vi "Config Input Type.vi"(0 "VISA resource name":refnum<visa-resource-name>, 1 "Sensor Type (0: Special)":i8(ring) items=["Special", "Silicon Diode", "GaAIAS Diode", "Platinum 100 (250 Ohm)", "Platinum 100 (500 Ohm)", "Platinum 1000", "Rhodium Iron", "Carbon Glass", "Cernox", "RuOx", "Germanium"], 2 "Coefficient (0: None)":i8(ring) items=["None", "Negative", "Positive"], 5 "Input (0: A)":u16(ring) items=["A", "B", "C", "D"], 7 "Units (0: None)":i8(ring) items=["None", "Volts", "Ohms"], 9 "Excitation (0: None)":i8(ring), 11 "error in (no error)":errorcluster, 12 "Range (0: None)":i8(ring) items=["None", "1mV", "2.5mV", "5mV", "10mV", "25mV", "50mV", "100mV", "250mV", "500mV", "1V", "2.5V", "5V", "7V"]) -> (4 "VISA resource name out":refnum<visa-resource-name>, 15 "error out":errorcluster)   [LabVIEW 2019, in "Lake Shore Cryotronics 340.lvlib"]
doc: "This VI configures the following parameters for a 340 input's type:\nSensor Type, Units, Coefficient, Excitation, and Range.\nNote that if Sensor Type is not special, none of the other parameters will not be sent as they are pre-determined by this instrument.\nThe LSCI 340 Status - Busy.vi should be used after this vi to verify the instrument has finished processing the commands."
uses:
  Lake Shore Cryotronics 340.lvlib
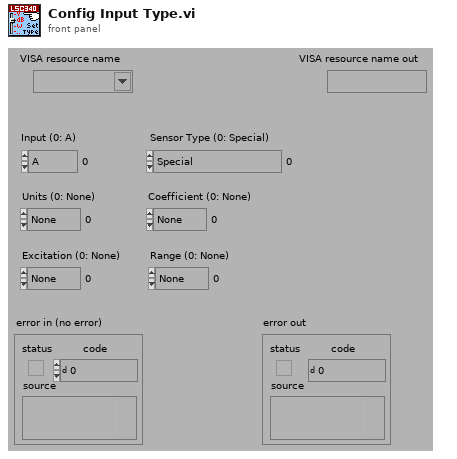
[diagram p1: front panel]
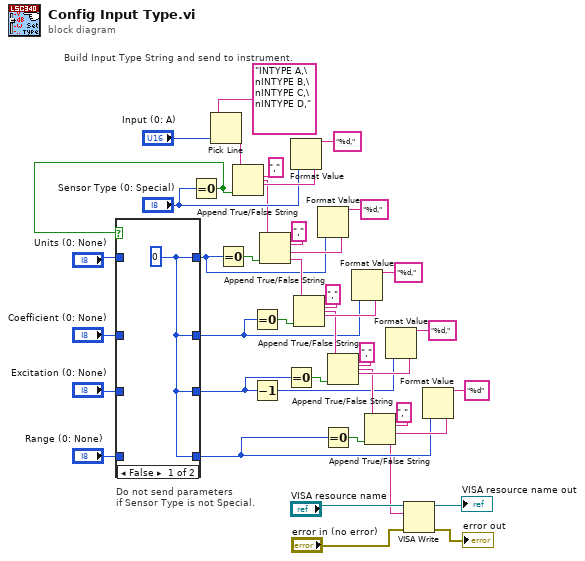
[diagram p0: block diagram]
diagram:
  # "Do not send parameters\nif Sensor Type is not Special."
  # "Build Input Type String and send to instrument."
  n1 = Equal To 0?(x="Sensor Type (0: Special)") -> (x = 0?=w14:bool)
  n2 = case shown="False" w14 {
    tunnel: [w43 w47] -> w13
    tunnel: [w43 w46] -> w12
    tunnel: [w43 w45] -> w11
    tunnel: [w43 w44] -> w10
    tunnel: "Units (0: None)" -> [_ w47]
    tunnel: "Coefficient (0: None)" -> [_ w46]
    tunnel: "Excitation (0: None)" -> [_ w45]
    tunnel: "Range (0: None)" -> [_ w44]
    frame False {
      w43 = 0
    }
    frame True {
    }
  }
  n3 = Pick Line(multi-line string="INTYPE A,\nINTYPE B,\nINTYPE C,\nINTYPE D,", line index="Input (0: A)") -> (output string=w40:string)  [unwired: 1 in]
  n4 = Equal To 0?(x=w13) -> (x = 0?=w35:bool)
  n5 = Equal To 0?(x=w12) -> (x = 0?=w30:bool)
  n6 = Decrement(x=w11) -> (x-1=w15:i32)
  n7 = Equal To 0?(x=w11) -> (x = 0?=w25:bool)
  n8 = Format Value(format string="%d,", value (0)="Sensor Type (0: Special)") -> (output string=w38:string)  [unwired: 1 in]
  n9 = Append True/False String(1:w14, 2:w38, 3:",", 4:w40) -> (0:w31:string)
  n10 = Format Value(format string="%d,", value (0)=w13) -> (output string=w33:string)  [unwired: 1 in]
  n11 = Append True/False String(1:w35, 2:w33, 3:",", 4:w31) -> (0:w26:string)
  n12 = Equal To 0?(x=w10) -> (x = 0?=w20:bool)
  n13 = Format Value(format string="%d,", value (0)=w12) -> (output string=w28:string)  [unwired: 1 in]
  n14 = Append True/False String(1:w30, 2:w28, 3:",", 4:w26) -> (0:w21:string)
  n15 = Format Value(format string="%d,", value (0)=w15) -> (output string=w23:string)  [unwired: 1 in]
  n16 = Append True/False String(1:w25, 2:w23, 3:",", 4:w21) -> (0:w16:string)
  n17 = Format Value(format string="%d", value (0)=w10) -> (output string=w18:string)  [unwired: 1 in]
  n18 = Append True/False String(1:w20, 2:w18, 3:",", 4:w16) -> (0:w1:string)
  n19 = VISA Write(VISA resource name="VISA resource name", write buffer=w1, error in (no error)="error in (no error)") -> (VISA resource name out=→"VISA resource name out":refnum<visa-resource-name>, error out=→"error out":errorcluster)  [unwired: 1 out]
